vi "Read 1d data.vi"(7 "Row Axis Path":string, 8 "error in (no error)":errorcluster, 10 "ModelManager":T1, 11 "Parameter Path":string) -> (0 "error out":errorcluster, 3 "TBL1D":cluster{"X":sgl[], "Y":sgl[]})   [LabVIEW 2011]
uses:
  <vilib>/NI Veristand/Execution/ModelManager/ModelManagerAPI.ctl
  NationalInstruments.VeriStand.ClientAPI
  <vilib>/NI Veristand/Execution/ModelManager/NI VeriStand - Get Parameter 2D Array Values.vi
  <vilib>/NI Veristand/Execution/ModelManager/NI_VS ModelManager ExecutionAPI.lvlib
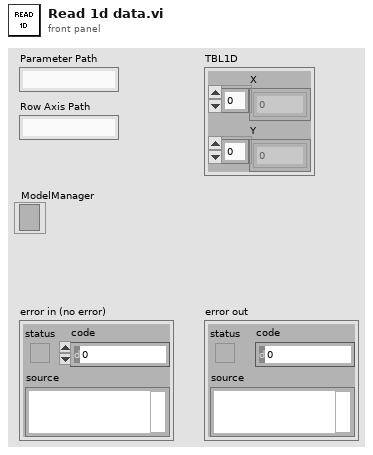
[diagram p1: front panel]
types:
  T1 = typedef "NI_VS ModelManager ExecutionAPI.lvlib/ModelManagerAPI.ctl" = refnum<k24>
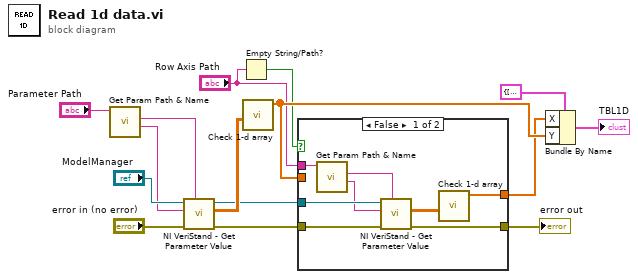
[diagram p0: block diagram]
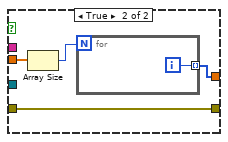
[diagram p2: hidden frame]
diagram:
  n1 = call "Get Param Path & Name.vi"("Path"="Parameter Path") -> ("Parameter Path"=w6:string, "Controller name"=w7:string)  [unwired: 8 in, 1 out]
  n2 = call-poly <vilib>:"NI VeriStand - Get Parameter Value.vi"("Target"=w7, "error in (no error)"="error in (no error)", "Parameter"=w6, "ModelManager in"="ModelManager") -> ("error out"=w4:errorcluster, "Values"=w9:dbl[][], "ModelManager out"=w5:T1)  [unwired: 5 in]
  n3 = Empty String/Path?(string/path="Row Axis Path") -> (empty?=w3:bool)
  n4 = call "Check 1-d array.vi"("Array"=w9) -> ("Array 2"=w14:dbl[])  [unwired: 10 in]
  n5 = case shown="False" w3 {
    tunnel: w14 -> [_ w27]
    tunnel: [w16 w26] -> w13
    tunnel: w5 -> [w23 _]
    tunnel: w4 -> [w22 w24]
    tunnel: "Row Axis Path" -> [w21 _]
    tunnel: [w18 w24] -> w1
    frame False {
      n6 = call "Get Param Path & Name.vi"("Path"=w21) -> ("Parameter Path"=w19:string, "Controller name"=w20:string)  [unwired: 8 in, 1 out]
      n7 = call-poly <vilib>:"NI VeriStand - Get Parameter Value.vi"("Target"=w20, "error in (no error)"=w22, "Parameter"=w19, "ModelManager in"=w23) -> ("error out"=w18:errorcluster, "Values"=w17:dbl[][])  [unwired: 5 in, 1 out]
      n8 = call "Check 1-d array.vi"("Array"=w17) -> ("Array 2"=w16:dbl[])  [unwired: 10 in]
    }
    frame True {
      n9 = Array Size(array=w27) -> (size(s)=w25:i32)
      n10 = for {
        N: w25 -> [_]
        tunnel: [w28] -> w26 mode=indexing
        i -> [w28]
      }
    }
  }
  "error out" <- w1
  n11 = Bundle By Name(cluster=cluster{"X":sgl[], "Y":sgl[]} {"X"=[0.0, 1.0, 2.0, 3.0], "Y"=[5.0, 0.0, 1.0, 5.0]} ("TBL1D"), "X"=w13, "Y"=w14) -> (→"TBL1D":cluster{"X":sgl[], "Y":sgl[]})
